vi "draw complex lorentzian.vi"(11 "4 corners":T1={"z (-pi/2)"=-1.0311345636926572+0.5736824521422934i, "z(inf)"=-0.5200164984937075+1.0975277942502903i, "z (pi/2)"=-1.0311345636926572+0.5736824521422934i, "z center"=-0.5136528600391839+0.580046090596817i, "z(0)"=-0.5200164984937075+1.0975277942502903i, "radius"=-1.0311345636926572}) -> (2 "fancy circles":cluster{dbl[], dbl[]}[](array[cluster]))   [LabVIEW 2018]
uses:
  circle corners.ctl
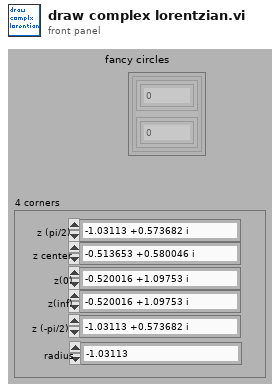
[diagram p1: front panel]
types:
  T1 = typedef "circle corners.ctl" = cluster{"z (-pi/2)":cdb, "z(inf)":cdb, "z (pi/2)":cdb, "z center":cdb, "z(0)":cdb, "radius":dbl}
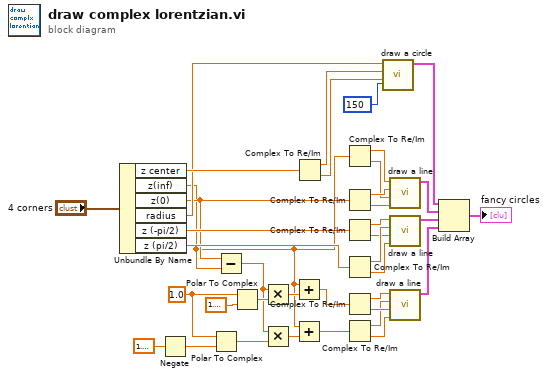
[diagram p0: block diagram]
diagram:
  w13 = 1.0 ("r")
  n1 = Unbundle By Name("4 corners") -> ("z center"=w21:cdb, "z(inf)"=w8:cdb, "z(0)"=w14:cdb, "radius"=w16:dbl, "z (-pi/2)"=w27:cdb, "z (pi/2)"=w26:cdb)
  n2 = Negate(x=1.5707963267948966) -> (-x=w17:dbl)
  n3 = Polar To Complex(1:w17, 2:w13) -> (0:w11:cdb)
  n4 = Subtract(x=w14, y=w8) -> (x-y=w12:cdb)
  n5 = Polar To Complex(1:1.5707963267948966, 2:w13) -> (0:w15:cdb)
  n6 = Multiply(x=w12, y=w15) -> (x*y=w10:cdb)
  n7 = Multiply(x=w12, y=w11) -> (x*y=w9:cdb)
  n8 = Add(x=w8, y=w10) -> (x+y=w7:cdb)
  n9 = Add(x=w8, y=w9) -> (x+y=w6:cdb)
  n10 = Complex To Re/Im(x + iy=w21) -> (x=w32:dbl, y=w33:dbl)
  n11 = Complex To Re/Im(x + iy=w8) -> (x=w37:dbl, y=w35:dbl)
  n12 = Complex To Re/Im(x + iy=w14) -> (x=w36:dbl, y=w34:dbl)
  n13 = Complex To Re/Im(x + iy=w27) -> (x=w31:dbl, y=w29:dbl)
  n14 = Complex To Re/Im(x + iy=w26) -> (x=w30:dbl, y=w28:dbl)
  n15 = Complex To Re/Im(x + iy=w7) -> (x=w5:dbl, y=w4:dbl)
  n16 = Complex To Re/Im(x + iy=w6) -> (x=w3:dbl, y=w2:dbl)
  n17 = call "draw a circle.vi"("number of points"=150, "center Y"=w33, "center x"=w32, "radius"=w16) -> ("output cluster"=w38:cluster{dbl[], dbl[]})  [unwired: 7 in]
  n18 = call "draw a line.vi"("y1"=w34, "y0"=w35, "x1"=w36, "x0"=w37) -> ("output cluster"=w25:cluster{dbl[], dbl[]})  [unwired: 7 in]
  n19 = call "draw a line.vi"("y1"=w28, "y0"=w29, "x1"=w30, "x0"=w31) -> ("output cluster"=w24:cluster{dbl[], dbl[]})  [unwired: 7 in]
  n20 = call "draw a line.vi"("y1"=w2, "y0"=w4, "x1"=w3, "x0"=w5) -> ("output cluster"=w1:cluster{dbl[], dbl[]})  [unwired: 7 in]
  n21 = Build Array(w38, w25, w24, w1) -> (→"fancy circles":cluster{dbl[], dbl[]}[])
